vi "SFCS_GetMAC.vi"() -> (0 "Status (NG or MAC address)":string)   [LabVIEW 2011]
uses:
  Instance           3 19Saved   SFCS_GetMAC .vi
  Instance           8 19Saved   SFCS_GetMAC .vi
  Instance           9 19Saved   SFCS_GetMAC .vi
  Instance          10 19Saved   SFCS_GetMAC .vi
  Instance          13 19Saved   SFCS_GetMAC .vi
  data/MCSDLL.dll
  Instance          16 19Saved   SFCS_GetMAC .vi
panel:
  out "軟體版本 Software Version":string
  out "begin time":u32
  out "IDTYPE":i32
  out "SN":string
  out "SeqNo":i32
  out "Sequence":string
  out "Category":string
  out "STAGE":string
  out "SFCS_IP":string
  out "Status":bool
  in  "URL":string
  # "Get MAC (SFCS_USNItem)"
  # "2014-8-6"
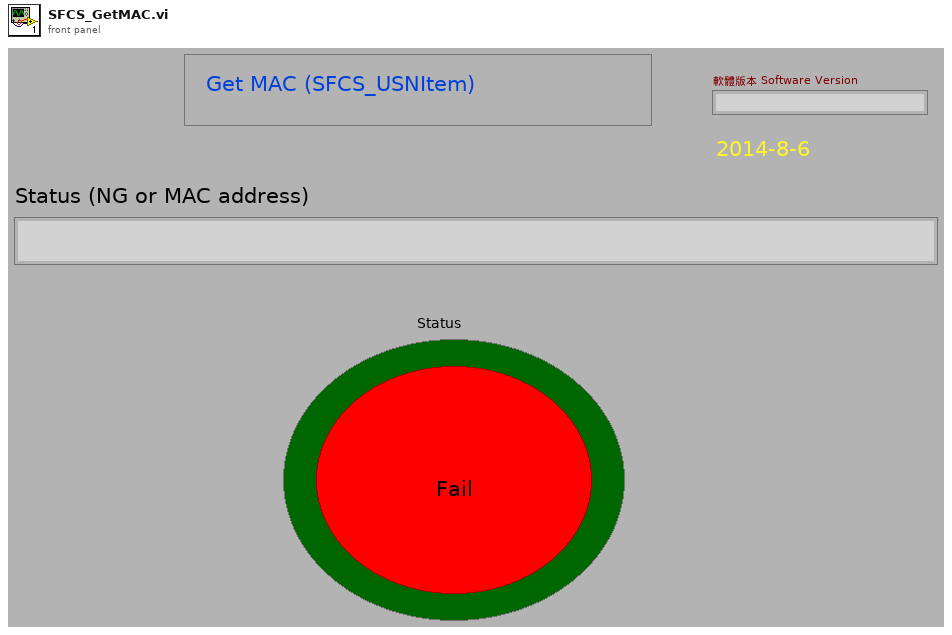
[diagram p1: front panel]
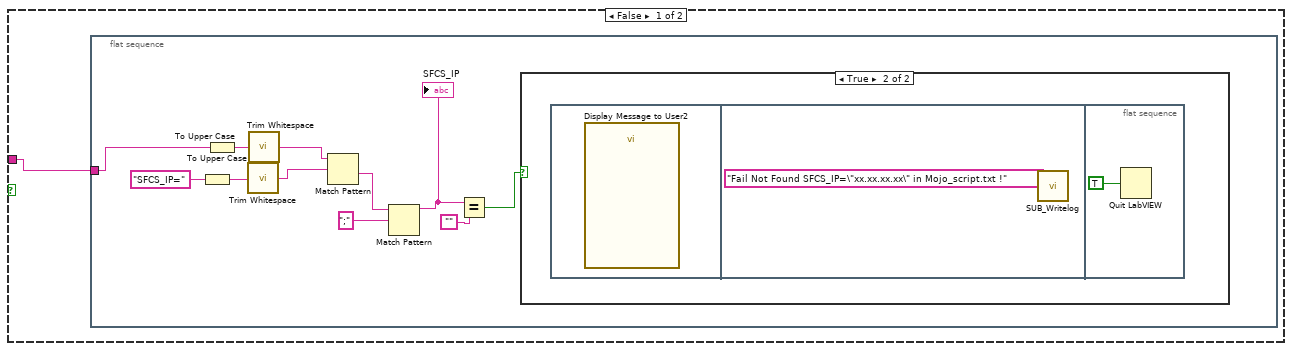
[diagram p3: hidden frame]
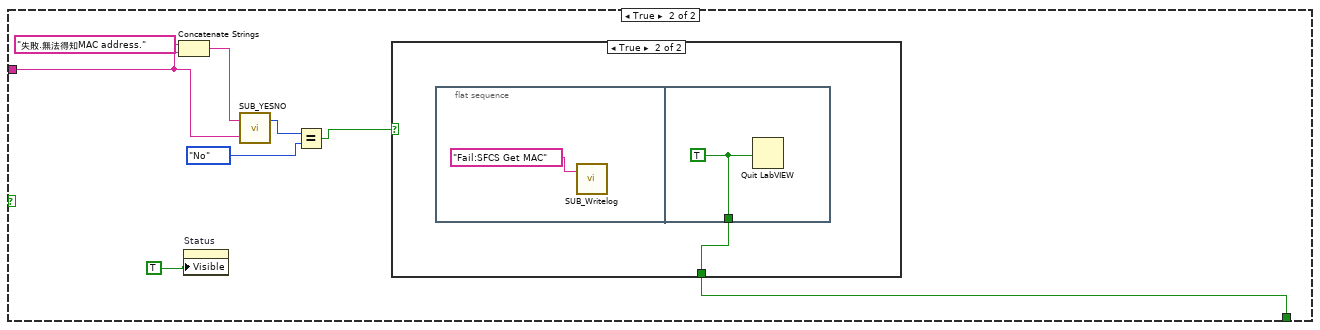
[diagram p8: hidden frame]
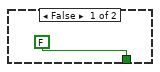
[diagram p9: hidden frame]
diagram:
  n1 = flat-sequence {
    tunnel: [w11] -> w1
    tunnel: w1 -> [w33]
    frame #0 {
      n2 = Tick Count (ms)() -> (millisecond timer value=→"begin time":u32)
    }
    frame #1 {
      n3 = property on="Status" class="Bool (strict)"("Visible"=FALSE) -> ()  [unwired: 2 in, 2 out]
    }
    frame #2 {
      n4 = call "SUB_SW_Version.vi"() -> ("Current Software Version"=→"軟體版本 Software Version":string)  [unwired: 3 in]
    }
    frame #3 {
      n5 = call "SUB_SearchFile_inFolder.vi"("Search Filename in Folder"="SFCS_INFO.LOG") -> ("File Existing True/Flase"=w5:bool)  [unwired: 1 in]
      n6 = case shown="False" w5 {
        frame False {
          n7 = flat-sequence {
            frame #0 {
              n8 = call "Display Message to User3"() -> ()  [unwired: 10 in, 2 out]
            }
            frame #1 {
              n9 = call "SUB_Writelog.vi"("Pass/Fail"="Fail :Please Do Check Route First !") -> ()  [unwired: 2 in]
            }
            frame #2 {
              n10 = Quit LabVIEW(quit? (T)=TRUE) -> ()
            }
          }
        }
        frame True {
        }
      }
    }
    frame #4 {
      n11 = call "SUB_DELETE_SpecificFile.vi"("Filename to be  Deleted"="PQAW_MAC.log") -> ()  [unwired: 2 in, 1 out]
    }
    frame #5 {
      n12 = call "SUB_Read_specifFile.vi"("name or relative path"="S8300E_sfcs_misc.txt" ("Script FileName")) -> ("error out"=w14:errorcluster, "text"=w11:string)  [unwired: 1 in]
      n13 = Unbundle By Name(w14) -> ("code"=w13:i32)
      n14 = Not Equal To 0?(x=w13) -> (x != 0?=w12:bool)
      n15 = case shown="True" w12 {
        tunnel: w11 -> [w15 _]
        frame False {
          n16 = flat-sequence {
            tunnel: w15 -> [w21]
            frame #0 {
              n17 = To Upper Case(1:"SFCS_IP=" ("string")) -> (0:w25:string)
              n18 = To Upper Case(1:w21) -> (0:w26:string)
              n19 = call <vilib>:"Trim Whitespace.vi"("string"=w25) -> ("trimmed string"=w23:string)  [unwired: 1 in]
              n20 = call <vilib>:"Trim Whitespace.vi"("string"=w26) -> ("trimmed string"=w22:string)  [unwired: 1 in]
              n21 = Match Pattern(string=w22, regular expression=w23) -> (after substring=w20:string)  [unwired: 1 in, 3 out]
              n22 = Match Pattern(string=w20, regular expression=";") -> (before substring=w18:string)  [unwired: 1 in, 3 out]
              "SFCS_IP" <- w18
              n23 = Equal?(x=w18, y="") -> (x = y?=w16:bool)
              n24 = case shown="True" w16 {
                frame False {
                }
                frame True {
                  n25 = flat-sequence {
                    frame #0 {
                      n26 = call "Display Message to User2"() -> ()  [unwired: 10 in, 2 out]
                    }
                    frame #1 {
                      n27 = call "SUB_Writelog.vi"("Pass/Fail"="Fail Not Found SFCS_IP=\"xx.xx.xx.xx\" in Mojo_script.txt !") -> ()  [unwired: 2 in]
                    }
                    frame #2 {
                      n28 = Quit LabVIEW(quit? (T)=TRUE) -> ()
                    }
                  }
                }
              }
            }
          }
        }
        frame True {
          n29 = flat-sequence {
            frame #0 {
              n30 = call "Display Message to User"() -> ()  [unwired: 10 in, 2 out]
            }
            frame #1 {
              n31 = call "SUB_Writelog.vi"("Pass/Fail"="Fail S8300E_sfcs_misc.txt is Missing!") -> ()  [unwired: 2 in]
            }
            frame #2 {
              n32 = Quit LabVIEW(quit? (T)=TRUE) -> ()
            }
          }
        }
      }
    }
    frame #6 {
      n33 = To Upper Case(1:"SFCS_ID_TYPE=" ("string")) -> (0:w39:string)
      n34 = To Upper Case(1:w33) -> (0:w40:string)
      n35 = call <vilib>:"Trim Whitespace.vi"("string"=w39) -> ("trimmed string"=w38:string)  [unwired: 1 in]
      n36 = call <vilib>:"Trim Whitespace.vi"("string"=w40) -> ("trimmed string"=w37:string)  [unwired: 1 in]
      n37 = To Upper Case(1:"SFCS_STAGE=" ("string")) -> (0:w72:string)
      n38 = To Upper Case(1:w33) -> (0:w73:string)
      n39 = To Upper Case(1:"SFCS_Category=" ("string")) -> (0:w65:string)
      n40 = To Upper Case(1:w33) -> (0:w66:string)
      n41 = Match Pattern(string=w37, regular expression=w38) -> (after substring=w36:string)  [unwired: 1 in, 3 out]
      n42 = call <vilib>:"Trim Whitespace.vi"("string"=w72) -> ("trimmed string"=w71:string)  [unwired: 1 in]
      n43 = call <vilib>:"Trim Whitespace.vi"("string"=w73) -> ("trimmed string"=w70:string)  [unwired: 1 in]
      n44 = To Upper Case(1:"SFCS_Sequence=" ("string")) -> (0:w58:string)
      n45 = call <vilib>:"Trim Whitespace.vi"("string"=w65) -> ("trimmed string"=w64:string)  [unwired: 1 in]
      n46 = call <vilib>:"Trim Whitespace.vi"("string"=w66) -> ("trimmed string"=w63:string)  [unwired: 1 in]
      n47 = To Upper Case(1:w33) -> (0:w59:string)
      n48 = Match Pattern(string=w36, regular expression=";") -> (before substring=w32:string)  [unwired: 1 in, 3 out]
      n49 = call <vilib>:"Trim Whitespace.vi"("string"=w58) -> ("trimmed string"=w57:string)  [unwired: 1 in]
      n50 = call <vilib>:"Trim Whitespace.vi"("string"=w59) -> ("trimmed string"=w56:string)  [unwired: 1 in]
      n51 = Match Pattern(string=w70, regular expression=w71) -> (after substring=w69:string)  [unwired: 1 in, 3 out]
      n52 = Match Pattern(string=w63, regular expression=w64) -> (after substring=w62:string)  [unwired: 1 in, 3 out]
      n53 = Decimal String To Number(string=w32) -> (number=→"IDTYPE":i32)  [unwired: 2 in, 1 out]
      n54 = Match Pattern(string=w56, regular expression=w57) -> (after substring=w55:string)  [unwired: 1 in, 3 out]
      n55 = Match Pattern(string=w69, regular expression=";") -> (before substring=w52:string)  [unwired: 1 in, 3 out]
      "STAGE" <- w52
      n56 = Match Pattern(string=w62, regular expression=";") -> (before substring=w51:string)  [unwired: 1 in, 3 out]
      "Category" <- w51
      n57 = Match Pattern(string=w55, regular expression=";") -> (before substring=w42:string)  [unwired: 1 in, 3 out]
      "Sequence" <- w42
      n58 = Decimal String To Number(string=w42) -> (number=→"SeqNo":i32)  [unwired: 2 in, 1 out]
      n59 = Not Equal?(x=w51, y="") -> (x != y?=w46:bool)
      n60 = Not Equal?(x=w52, y="") -> (x != y?=w47:bool)
      n61 = Not Equal?(x=w42, y="") -> (x != y?=w44:bool)
      n62 = And(x=w47, y=w46) -> (x .and. y?=w45:bool)
      n63 = And(x=w45, y=w44) -> (x .and. y?=w43:bool)
      n64 = case shown="False" w43 {
        frame False {
          n65 = flat-sequence {
            frame #0 {
              n66 = call "Display Message to User4"() -> ()  [unwired: 10 in, 2 out]
            }
            frame #1 {
              n67 = call "SUB_Writelog.vi"("Pass/Fail"="Fail :Stage,Category,Sequence not define in script file!") -> ()  [unwired: 2 in]
            }
            frame #2 {
              n68 = Quit LabVIEW(quit? (T)=TRUE) -> ()
            }
          }
        }
        frame True {
        }
      }
    }
    frame #7 {
      n69 = call "SUB_Read_specifFile.vi"("name or relative path"="SFCS_INFO.LOG") -> ("error out"=w86:errorcluster, "text"=w85:string)  [unwired: 1 in]
      n70 = Unbundle By Name(w86) -> ("code"=w83:i32)
      n71 = call "SUB_FindSpecificString.vi"("Find this String"="USN=", "String data"=w85) -> ("before \"; \" string"=→"SN":string, "Found"=w81:bool)  [unwired: 2 in]
      n72 = Equal?(x=w83, y=0) -> (x = y?=w78:bool)
      n73 = Equal?(x=w81, y=TRUE) -> (x = y?=w79:bool)
      n74 = And(x=w79, y=w78) -> (x .and. y?=w76:bool)
      n75 = case shown="False" w76 {
        frame False {
          n76 = flat-sequence {
            frame #0 {
              n77 = call "Display Message to User5"() -> ()  [unwired: 10 in, 2 out]
            }
            frame #1 {
              n78 = call "SUB_Writelog.vi"("Pass/Fail"="Fail :Something is wrong in SFCS_INFO.LOG") -> ()  [unwired: 2 in]
            }
            frame #2 {
              n79 = Quit LabVIEW(quit? (T)=TRUE) -> ()
            }
          }
        }
        frame True {
        }
      }
    }
    frame #8 {
      n80 = local write "Status"(FALSE ("Status")) -> ()
    }
    frame #9 {
      n81 = local read "SFCS_IP"() -> (w91:string)
      n82 = local write "URL"(w91) -> ()
      n83 = local write "Status (NG or MAC address)"("") -> ()
    }
    frame #10 {
      n84 = while {
        stop <- w98 stop-if-true
        n85 = local read "STAGE"() -> (w100:string)
        n86 = local read "SN"() -> (w101:string)
        n87 = local read "IDTYPE"() -> (w99:i32)
        n88 = local read "SeqNo"() -> (w102:i32)
        n89 = dll-call lib="D:/S8300E_Project/data/MCSDLL.dll" fn="SFCS_GetUsnID"("URL"="URL", "SN"=w101, "Stage"=w100, "IDTYPE"=w99, "Sequence"=w102) -> (w107:string)  [unwired: 8 in, 2 out]
        "Status (NG or MAC address)" <- w107
        n90 = To Upper Case(1:"NG" ("string")) -> (0:w111:string)
        n91 = To Upper Case(1:w107) -> (0:w112:string)
        n92 = call <vilib>:"Trim Whitespace.vi"("string"=w111) -> ("trimmed string"=w108:string)  [unwired: 1 in]
        n93 = call <vilib>:"Trim Whitespace.vi"("string"=w112) -> ("trimmed string"=w106:string)  [unwired: 1 in]
        n94 = String Length(string=w106) -> (length=w95:i32)
        n95 = Match Pattern(string=w106, regular expression=w108) -> (match substring=w109:string)  [unwired: 1 in, 3 out]
        n96 = Not Equal?(x=w95, y=12) -> (x != y?=w94:bool)
        n97 = Not Equal?(x=w95, y=17) -> (x != y?=w93:bool)
        n98 = Equal?(x=w109, y=w108) -> (x = y?=w104:bool)
        n99 = Not Exclusive Or(1:w93, 2:w94) -> (0:w97:bool)
        n100 = Or(x=w97, y=w104) -> (x .or. y?=w103:bool)
        n101 = case shown="False" w103 {
          tunnel: w107 -> [w117 w143]
          tunnel: [w115 w142] -> w98
          frame False {
            n102 = flat-sequence {
              tunnel: w117 -> [w120]
              tunnel: [w120] -> w116
              tunnel: w116 -> [w127]
              tunnel: [w126] -> w114
              tunnel: w114 -> [w132]
              tunnel: [w141] -> w115
              frame #0 {
                n103 = local write "Status"(TRUE ("Status")) -> ()
                n104 = property on="Status" class="Bool (strict)"("Visible"=TRUE) -> ()  [unwired: 2 in, 2 out]
              }
              frame #1 {
                n105 = call <vilib>:"Trim Whitespace.vi"("string"=w127) -> ("trimmed string"=w125:string)  [unwired: 1 in]
                n106 = To Upper Case(1:w125) -> (0:w122:string)
                n107 = Concatenate Strings("Get  MAC from system=", w127) -> (w126:string)
                n108 = Concatenate Strings("LAN_MAC=", w122, ";") -> (w124:string)
                n109 = call "SUB_WriteMAC_toFile.vi"("MAC Address"=w124) -> ()  [unwired: 2 in]
              }
              frame #2 {
                w131 = "\n"
                n110 = local read "begin time"() -> (w136:u32)
                n111 = Tick Count (ms)() -> (millisecond timer value=w135:u32)
                n112 = call "SUB_CAL_TESTTIME.vi"("Test Item name"="SFCS_GetMAC", "Stop tick time"=w135, "Start tick time"=w136) -> ("Test Time output"=w130:string)  [unwired: 2 in]
                n113 = Concatenate Strings("Pass : SFCS_GETMAC" ("Pass/Fail"), w131, w132, w131, w130) -> (w129:string)
                n114 = call "SUB_Writelog.vi"("Pass/Fail"=w129) -> ()  [unwired: 2 in]
              }
              frame #3 {
                n115 = case shown="True" FALSE {
                  frame False {
                  }
                  frame True {
                    n116 = local read "Status (NG or MAC address)"() -> (w139:string)
                    n117 = Concatenate Strings("從系統的訊息" ("string"), w139) -> (w138:string)
                    n118 = call "Display Message to User6"("Message"=w138) -> ()  [unwired: 9 in, 2 out]
                  }
                }
              }
              frame #4 {
                w141 = TRUE ("quit? (T)")
                n119 = Quit LabVIEW(quit? (T)=w141) -> ()
              }
            }
          }
          frame True {
            n120 = Concatenate Strings("失敗.無法得知MAC address." ("string"), w143) -> (w144:string)
            n121 = property on="Status" class="Bool (strict)"("Visible"=TRUE) -> ()  [unwired: 2 in, 2 out]
            n122 = call "SUB_YESNO.vi"("Debug View"=w143, "Status"=w144) -> ("yes/no"=w149:enum32{"No Selection", "Yes", "No", "None"})  [unwired: 1 in]
            n123 = Equal?(x=w149, y=enum32{"No Selection", "Yes", "No", "None"}."No") -> (x = y?=w147:bool)
            n124 = case shown="True" w147 {
              tunnel: [FALSE w151] -> w142
              frame False {
              }
              frame True {
                n125 = flat-sequence {
                  tunnel: [w153] -> w151
                  frame #0 {
                    n126 = call "SUB_Writelog.vi"("Pass/Fail"="Fail:SFCS Get MAC") -> ()  [unwired: 2 in]
                  }
                  frame #1 {
                    w153 = TRUE
                    n127 = Quit LabVIEW(quit? (T)=w153) -> ()
                  }
                }
              }
            }
          }
        }
      }
    }
  }
